vi "Differential_Drive_Kinematics.vi"(8 "Scale_Down_For_Turn":bool, 9 "Angular_Throttle":dbl, 10 "Linear_Throttle":dbl) -> (1 "Right_Motor_Velocity(rotations/s)":dbl, 2 "Left_Motor_Velocity(rotations/s)":dbl)   [LabVIEW 2019]
panel:
  in  "Gear_Reduction(output/input)":dbl
  in  "Wheel_Base_Radius(in)":dbl
  in  "Wheel_Radius(in)":dbl
  in  "Max_Angular_Speed(rad/s)":dbl
  in  "Max_Linear_Speed(in/s)":dbl
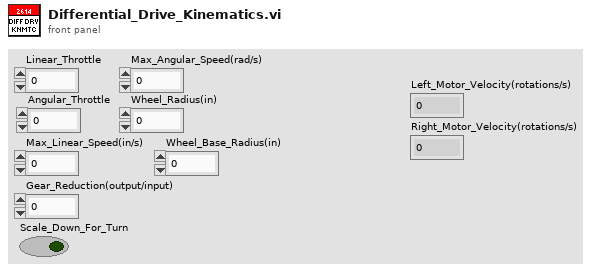
[diagram p1: front panel]
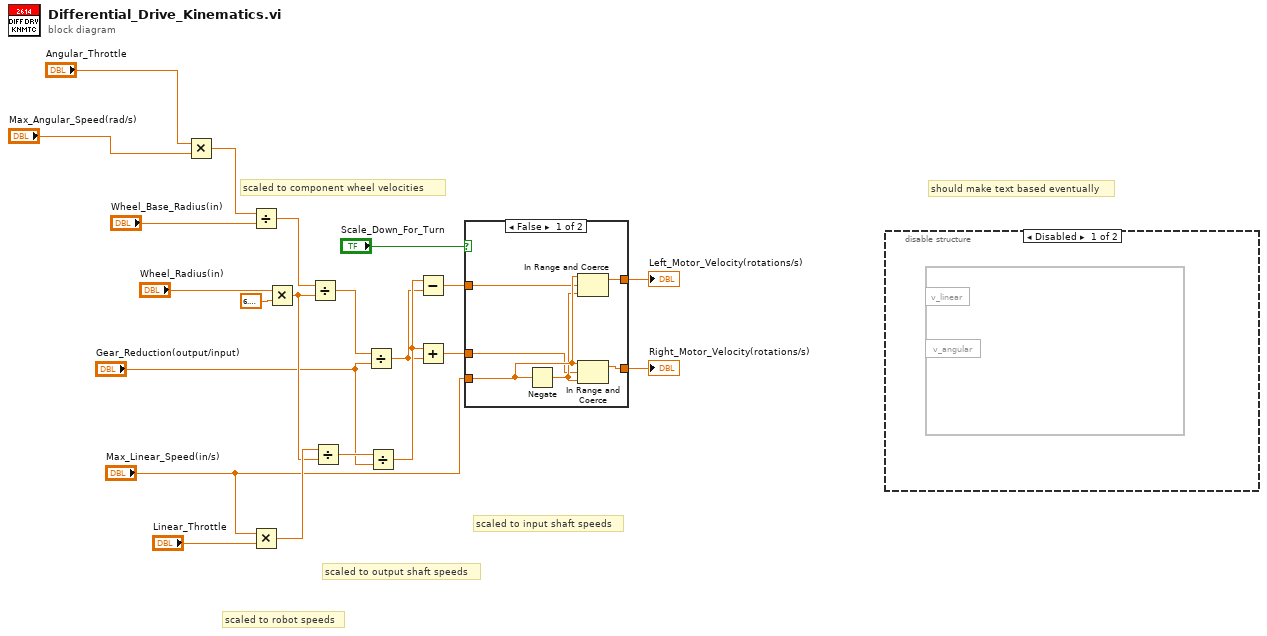
[diagram p0: block diagram]
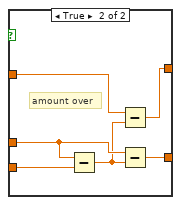
[diagram p3: hidden frame]
diagram:
  # "should make text based eventually"
  # "scaled to component wheel velocities"
  # "scaled to input shaft speeds"
  # "scaled to output shaft speeds"
  # "scaled to robot speeds"
  n1 = Multiply(x="Angular_Throttle", y="Max_Angular_Speed(rad/s)") -> (x*y=w14:dbl)
  n2 = Divide(x=w14, y="Wheel_Base_Radius(in)") -> (x/y=w12:dbl)
  n3 = Multiply(x="Max_Linear_Speed(in/s)", y="Linear_Throttle") -> (x*y=w16:dbl)
  n4 = Multiply(x="Wheel_Radius(in)", y=6.283185307179586) -> (x*y=w11:dbl)
  n5 = Divide(x=w12, y=w11) -> (x/y=w10:dbl)
  n6 = Divide(x=w16, y=w11) -> (x/y=w15:dbl)
  n7 = Divide(x=w10, y="Gear_Reduction(output/input)") -> (x/y=w7:dbl)
  n8 = Divide(x=w15, y="Gear_Reduction(output/input)") -> (x/y=w8:dbl)
  n9 = Subtract(x=w8, y=w7) -> (x-y=w4:dbl)
  n10 = Add(x=w8, y=w7) -> (x+y=w3:dbl)
  n11 = case shown="False" "Scale_Down_For_Turn" {
    tunnel: "Max_Linear_Speed(in/s)" -> [w27 w33]
    tunnel: w4 -> [w25 w30]
    tunnel: w3 -> [w24 w31]
    tunnel: [w23 w32] -> w2
    tunnel: [w22 w28] -> w1
    frame False {
      n12 = Negate(x=w27) -> (-x=w26:dbl)
      n13 = In Range and Coerce(upper limit=w27, x=w25, lower limit=w26) -> (coerced(x)=w22:dbl)  [unwired: 1 out]
      n14 = In Range and Coerce(upper limit=w27, x=w24, lower limit=w26) -> (coerced(x)=w23:dbl)  [unwired: 1 out]
    }
    frame True {
      # "amount over"
      n15 = Subtract(x=w31, y=w33) -> (x-y=w29:dbl)
      n16 = Subtract(x=w30, y=w29) -> (x-y=w28:dbl)
      n17 = Subtract(x=w31, y=w29) -> (x-y=w32:dbl)
    }
  }
  "Right_Motor_Velocity(rotations/s)" <- w2
  "Left_Motor_Velocity(rotations/s)" <- w1
  n18 = disable-structure shown="Disabled" {
    frame Disabled {
      n19 = formula code=""() -> ()  [unwired: 2 in]
    }
    frame Enabled {
    }
  }
